vi "get work space cycles.vi"(11 "which position to view":string) -> (3 "transposed array":dbl[][](array[numeric]))   [LabVIEW 2016]
uses:
  controls/cycle results control.ctl
panel:
  out "cycle results cluster out":T1
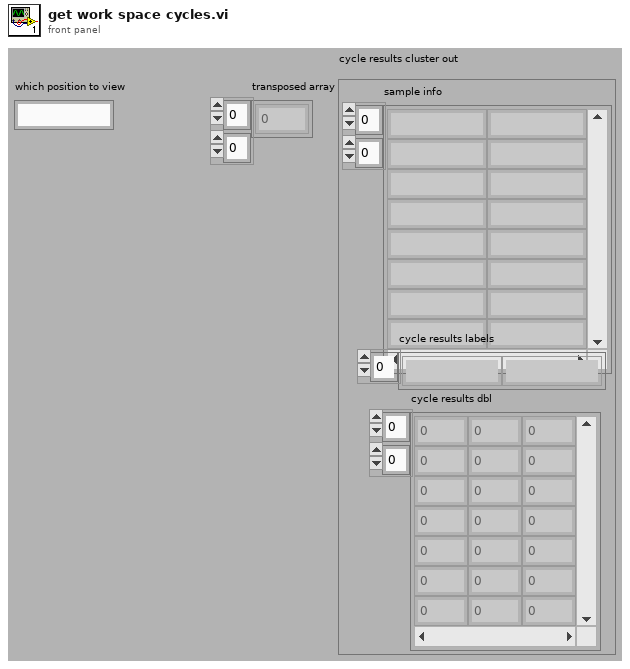
[diagram p1: front panel]
types:
  T1 = typedef "cycle results control.ctl" = cluster{"sample info":string[][], "cycle results labels":string[], "cycle results dbl":dbl[][]}
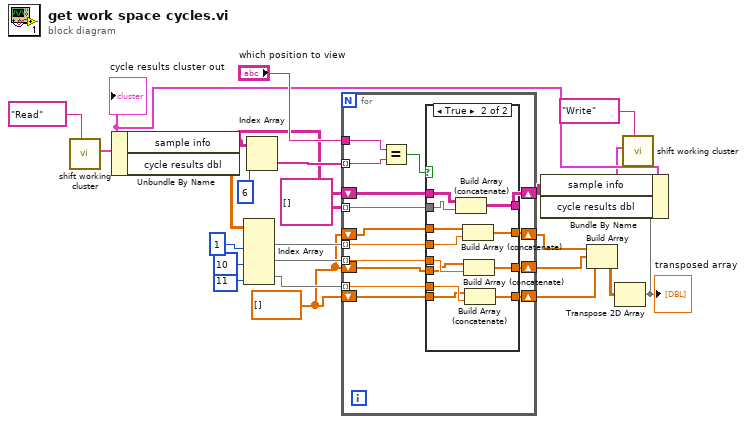
[diagram p0: block diagram]
diagram:
  w6 = dbl[] []
  n1 = call "shift working cluster.vi"("read write shift"="Read") -> ("cycle results cluster out"=w15:T1)  [unwired: 9 in, 1 out]
  "cycle results cluster out" <- w15
  n2 = Unbundle By Name(w15) -> ("sample info"=w18:string[][], "cycle results dbl"=w12:dbl[][])
  n3 = Index Array(array=w12, index (col) #1=1 ("disabled index (col)"), index (col) #2=10 ("index (col)"), index (col) #3=11 ("index (col)")) -> (element #1=w10:dbl[], element #2=w9:dbl[], element #3=w7:dbl[])  [unwired: 3 in]
  n4 = Index Array(array=w18, index (col)=6 ("disabled index (col)")) -> (element=w20:string[])  [unwired: 1 in]
  n5 = for {
    tunnel: w20 -> [w38] mode=indexing
    tunnel: "which position to view" -> [w37]
    tunnel: w18 -> [w35] mode=indexing
    shift-right: [w34] -> w16
    shift-left: string[][] [] -> [w33]
    tunnel: w10 -> [w32] mode=indexing
    tunnel: w9 -> [w31] mode=indexing
    shift-right: [w30] -> w4
    shift-left: w6 -> [w24]
    shift-right: [w29] -> w5
    shift-left: w6 -> [w28]
    tunnel: w7 -> [w27] mode=indexing
    shift-right: [w26] -> w3
    shift-left: w6 -> [w25]
    n6 = Equal?(x=w37, y=w38) -> (x = y?=w36:bool)
    n7 = case shown="True" w36 {
      tunnel: w35 -> [_ w54]
      tunnel: [w42 w53] -> w34
      tunnel: w33 -> [w42 w52]
      tunnel: w32 -> [_ w51]
      tunnel: w31 -> [_ w50]
      tunnel: [w40 w49] -> w30
      tunnel: [w41 w48] -> w29
      tunnel: w28 -> [w41 w47]
      tunnel: w27 -> [_ w46]
      tunnel: [w39 w45] -> w26
      tunnel: w25 -> [w39 w44]
      tunnel: w24 -> [w40 w43]
      frame False {
      }
      frame True {
        n8 = Build Array (concatenate)(w52, w54) -> (w53:string[][])
        n9 = Build Array (concatenate)(w47, w51) -> (w48:dbl[])
        n10 = Build Array (concatenate)(w43, w50) -> (w49:dbl[])
        n11 = Build Array (concatenate)(w44, w46) -> (w45:dbl[])
      }
    }
  }
  n12 = Build Array(w5, w4, w3) -> (w2:dbl[][])
  n13 = Transpose 2D Array(2D array=w2) -> (transposed array=w1:dbl[][])
  "transposed array" <- w1
  n14 = Bundle By Name(cluster=w15, "sample info"=w16, "cycle results dbl"=w1) -> (w14:T1)
  n15 = call "shift working cluster.vi"("read write shift"="Write", "cycle results cluster In"=w14) -> ()  [unwired: 8 in, 2 out]
